vi "Image_Snap_Dual.vi"(8 "error in":errorcluster, 10 "input cluster":T1={"system"={"info"={"menuSelect"=0, "version"=0, "serial"="Test Sample", "captureActive"=TRUE, "captureBegin"=TRUE, "emptyAndRefill"=TRUE}, "userInfo"={"operatorName"="", "date"=timestamp(2713993200 s since 1904-01-01)}, "camera"={"exposureTime"=0, "aperture"=enum."Item 0", "framerate"=0, "framerateMax"=500, "legacyAttributes"=TRUE}}, "connections"={"arduino"={"connection"="First test samples", "status"=TRUE, "openState"=FALSE, "emptyStart"=0}, "pump"={"connection"="MRJ", "status"=TRUE, "command"="", "dispenseSpeed"=100, "flushSize"=100}, "camera"={"cam1"={"connection"="", "status"=FALSE}, "cam2"={"connection"="", "status"=FALSE}}}, "queue"={"process"={"cam1"=refnum, "cam2"=refnum, "queueSize"=0}, "save"={"cam1"=refnum, "cam2"=refnum, "queueSize"=0}, "overloadThreshold"=0}, "imageProcess"={"cam1"={"preAllocation"={"image"="Station", "originalDisplay"="Station", "originalRgb"="Station", "binary"="Station", "save"="Station", "calibrationFull"="remote image 0000000015E6FBB4", "calibrationDetect"="remote image 0000000015E6F134"}, "calibration"={"pathFull"=path "C:/Users/au540322/Desktop/IHS_Project/calibration/Test Calibration/Test Calibration_7/1Test Calibration_7_2019_06_07-23-38-32-452.PNG", "pathDetect"=path "C:/Users/au540322/Desktop/IHS_Project/calibration/Test Calibration/Test Calibration_7/2Test Calibration_7_2019_06_07-23-38-32-415.PNG", "ROI"={"Left"=0, "Top"=0, "Right"=0, "Bottom"=0, "Rotation"=0.0}}}, "cam2"={"preAllocation"={"image"=refnum, "originalDisplay"=refnum, "originalRgb"=refnum, "binary"=refnum, "save"=refnum, "calibrationFull"=refnum, "calibrationDetect"=refnum}, "calibration"={"pathFull"=path "C:/Users/au540322/Desktop/IHS_Project/images/Debris/Debris_0/Debris_0_2019_06_01-23-32-49-686.PNG", "pathDetect"=path "C:/Users/au540322/Desktop/IHS_Project/images/Debris/Debris_0/Debris_0_2019_06_01-23-32-49-686.PNG", "ROI"={"Left"=0, "Top"=0, "Right"=0, "Bottom"=0, "Rotation"=0.0}}}, "process"={"planeExtract"=refnum, "planeSubtract"=refnum, "cropMask"=refnum}, "detection"={"sampleTimeout"=500, "sizeThreshold"=500, "detectionRegionPct"=0.0}}, "sampleData"={"sampleId"="", "projectId"="", "voucherID"="", "speciesName"="", "collectionDate"=timestamp(2713993200 s since 1904-01-01), "sampleStation"="", "location"="", "lat"=0.0, "lon"=0.0, "determiner"="", "sex"="", "otherNotes"=""}, "Session In"=""} {"sampleData"."collectionDate" format="%<%Y-%m-%d>T"; "imageProcess"."detection"."sizeThreshold" min=1; "imageProcess"."cam2"."calibration"."ROI"."Rotation" format="%.2f"; "imageProcess"."cam2"."calibration"."ROI"."Left" scale=0.0..1024.0; "imageProcess"."cam2"."calibration"."ROI"."Right" scale=0.0..1024.0; "imageProcess"."cam1"."calibration"."ROI"."Rotation" format="%.2f"; "imageProcess"."cam1"."calibration"."ROI"."Left" scale=0.0..1024.0; "imageProcess"."cam1"."calibration"."ROI"."Right" scale=0.0..1024.0; "queue"."overloadThreshold" min=1; "queue"."save"."queueSize" min=1; "queue"."process"."queueSize" min=1; "connections"."pump"."flushSize" min=1; "connections"."pump"."dispenseSpeed" min=1; "system"."camera"."framerateMax" min=1; "system"."userInfo"."date" format="%<%Y-%m-%dT%H:%M:%S+%z>T"; "system"."info"."version" items=["Standard", "XL"]; "system"."info"."menuSelect" items=["Session Data", "Extended Setup", "Buffer", "Camera", "Dispenser", "Stats", "Connections"]}, 11 "Detect Movement":bool) -> (0 "error out":errorcluster, 1 "Image2":T3, 2 "Image1":T3, 3 "Framerate":i32)   [LabVIEW 2022 SP3]
doc: "Gather pictures from both cameras, returns two picture arrays."
uses:
  <vilib>/vision/Image Controls.llb/IMAQ Image.ctl
  controls/Data.ctl
  <vilib>/userdefined/High Color/IMAQdx.ctl
  <vilib>/vision/driver/IMAQdx.llb/IMAQdx Acquisition Mode.ctl
  Camera_ID.ctl
  <vilib>/vision/driver/NI_Vision_Acquisition_Software.lvlib
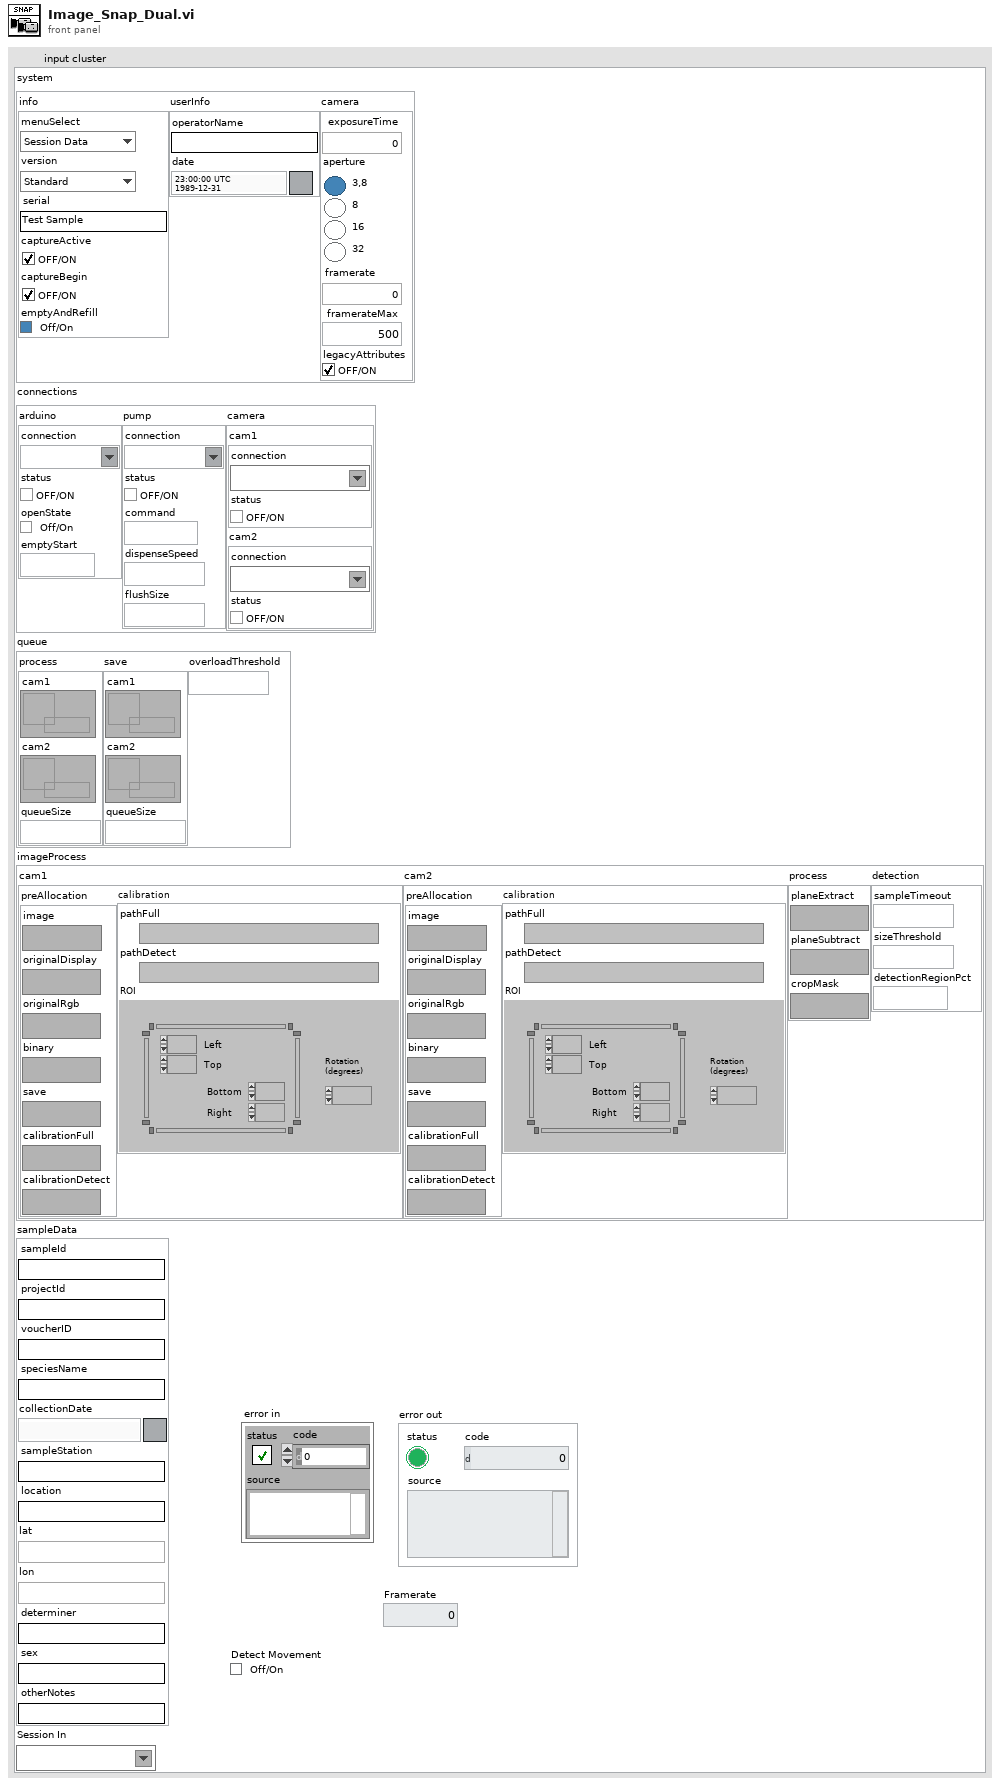
[diagram p1: front panel]
types:
  T1 = typedef "Data.ctl" = cluster{"system":cluster{"info":cluster{"menuSelect":u16, "version":u16, "serial":string, "captureActive":bool, "captureBegin":bool, "emptyAndRefill":bool}, "userInfo":cluster{"operatorName":string, "date":timestamp}, "camera":cluster{"exposureTime":i32, "aperture":enum32{"Item 0", "Item 1", "Item 2", "Item 3"}, "framerate":i32, "framerateMax":i32, "legacyAttributes":bool}}, "connections":cluster{"arduino":cluster{"connection":refnum<visa-resource-name>, "status":bool, "openState":bool, "emptyStart":u32}, "pump":cluster{"connection":refnum<visa-resource-name>, "status":bool, "command":string, "dispenseSpeed":i32, "flushSize":i32}, "camera":cluster{"cam1":cluster{"connection":T2, "status":bool}, "cam2":cluster{"connection":T2, "status":bool}}}, "queue":cluster{"process":cluster{"cam1":refnum<queue>, "cam2":refnum<queue>, "queueSize":i32}, "save":cluster{"cam1":refnum<queue>, "cam2":refnum<queue>, "queueSize":i32}, "overloadThreshold":i32}, "imageProcess":cluster{"cam1":cluster{"preAllocation":cluster{"image":T3, "originalDisplay":T3, "originalRgb":T3, "binary":T3, "save":T3, "calibrationFull":T3, "calibrationDetect":T3}, "calibration":cluster{"pathFull":path, "pathDetect":path, "ROI":T4}}, "cam2":cluster{"preAllocation":cluster{"image":T3, "originalDisplay":T3, "originalRgb":T3, "binary":T3, "save":T3, "calibrationFull":T3, "calibrationDetect":T3}, "calibration":cluster{"pathFull":path, "pathDetect":path, "ROI":T4}}, "process":cluster{"planeExtract":T3, "planeSubtract":T3, "cropMask":T3}, "detection":cluster{"sampleTimeout":i32, "sizeThreshold":i32, "detectionRegionPct":dbl}}, "sampleData":cluster{"sampleId":string, "projectId":string, "voucherID":string, "speciesName":string, "collectionDate":timestamp, "sampleStation":string, "location":string, "lat":dbl, "lon":dbl, "determiner":string, "sex":string, "otherNotes":string}, "Session In":T2}
  T2 = typedef "IMAQdx.ctl" = refnum<k21>
  T3 = typedef "IMAQ Image.ctl" = refnum<image>
  T4 = typedef "IMAQ Rectangle" = cluster{"Left":i32, "Top":i32, "Right":i32, "Bottom":i32, "Rotation":dbl}
  T5 = typedef "NI_Vision_Acquisition_Software.lvlib/IMAQdx Acquisition Mode.ctl" = enum32{"One Shot", "Continuous"}
  T6 = typedef "Camera_ID.ctl" = enum16{"Camera 1", "Camera 2"}
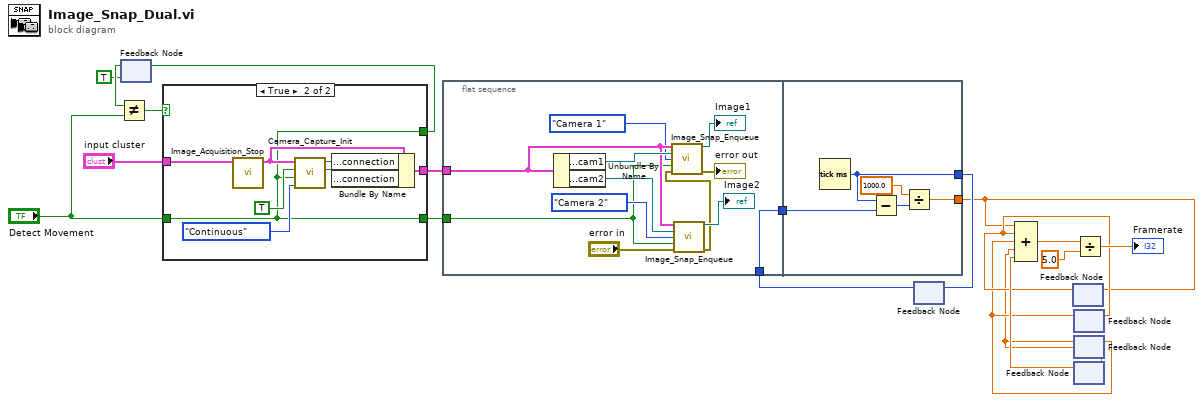
[diagram p0: block diagram]
diagram:
  n1 = feedback #1(TRUE ("Detect Movement")) -> (w5:bool)
  n2 = Not Equal?(x=w5, y="Detect Movement") -> (x != y?=w6:bool)
  n3 = case shown="True" w6 {
    tunnel: "input cluster" -> [w21 w22]
    tunnel: "Detect Movement" -> [w20 w23]
    tunnel: [w20 w23] -> w4
    tunnel: [w21 w24] -> w3
    tunnel: [w20 w23] -> w2
    frame False {
    }
    frame True {
      n4 = call "Image_Acquisition_Stop.vi"("input cluster"=w22) -> ("output cluster"=w25:T1)  [unwired: 9 in, 1 out]
      n5 = call "Camera_Capture_Init.vi"("Continuous?"=IMAQdx_Acquisition_Mode."Continuous", "Detect Movement"=w23, "Crop?"=TRUE, "input cluster"=w25) -> ("Camera2"=w26:T2, "Camera1"=w27:T2)  [unwired: 6 in]
      n6 = Bundle By Name(cluster=w25, "connections.camera.cam1.connection"=w27, "connections.camera.cam2.connection"=w26) -> (w24:T1)
    }
  }
  n7 = feedback-in #1(w4) -> ()
  n8 = flat-sequence {
    tunnel: [w34] -> w19
    tunnel: w17 -> [w34]
    tunnel: w3 -> [w33]
    tunnel: w2 -> [w30]
    tunnel: w19 -> [w46]
    tunnel: [w45] -> w18
    tunnel: [w42] -> w9
    frame #0 {
      n9 = Unbundle By Name(w33) -> ("queue.process.cam1"=w37:refnum<queue>, "queue.process.cam2"=w36:refnum<queue>)
      n10 = call "Image_Snap_Enqueue.vi"("input cluster"=w33, "Camera queue"=w36, "Camera"=Camera_ID."Camera 2", "Detect Movement"=w30, "error in"="error in") -> ("Image out"=→"Image2":T3, "error out"=w35:errorcluster)  [unwired: 9 in]
      n11 = call "Image_Snap_Enqueue.vi"("input cluster"=w33, "Camera queue"=w37, "Camera"=Camera_ID."Camera 1", "Detect Movement"=w30, "error in"=w35) -> ("Image out"=→"Image1":T3, "error out"=→"error out":errorcluster)  [unwired: 9 in]
    }
    frame #1 {
      n12 = Tick Count (ms)() -> (millisecond timer value=w45:u32)
      n13 = Subtract(x=w45, y=w46) -> (x-y=w44:u32)
      n14 = Divide(x=1000.0, y=w44) -> (x/y=w42:dbl)
    }
  }
  n15 = feedback #2() -> (w17:u32)  [unwired: 1 in]
  n16 = feedback-in #2(w18) -> ()
  n17 = feedback #3() -> (w12:dbl)  [unwired: 1 in]
  n18 = feedback-in #3(w9) -> ()
  n19 = feedback #4() -> (w11:dbl)  [unwired: 1 in]
  n20 = feedback-in #4(w12) -> ()
  n21 = feedback #5() -> (w10:dbl)  [unwired: 1 in]
  n22 = feedback-in #5(w11) -> ()
  n23 = feedback #6() -> (w13:dbl)  [unwired: 1 in]
  n24 = Compound Arithmetic op=ADD(w9, w12, w11, w10, w13) -> (w16:dbl)
  n25 = feedback-in #6(w10) -> ()
  n26 = Divide(x=w16, y=5.0) -> (x/y=→"Framerate":dbl)
